vi "001_Faith FT6400 Series.vi"(11 "Queue Ref":T1={"UI"=refnum, "Message"=refnum, "Data"=refnum, "Caller"=refnum, "Name"="000 Common", "Data Path"=path "D:/NBT/01-Project/02-Processing/NBT-TestPlatform V2/NBT-TestPlatform V2.0.3/Config/NBT/NBT_V1.0.0/Project/0001_HZKD_ST01/00_DataSource/001_PLC/01_PLC", "Class Path"=path "", "SubPanel"=refnum, "Project Name"="", "MNT"="", "Title"="", "Data Source"=refnum, "Queue List"={}, "VI"=refnum, "UE"=refnum}) -> ()   [LabVIEW 2020]
doc: "000001"
uses:
  Alin/QMH/000 Module Data Type.ctl
  Alin/QMH/Queue Message.ctl
  0007 Controls/005 Data Source Type.ctl
  9999 SubVI/Global/Data Global/SDQ Data Type.ctl
  002 Driver/002 Electronic Load/Load Param.ctl
  c9d39cc7-6b3d-4d6b-ac97-2b41707d41b7.vi
panel:
  out "QN":i32
  in  "Panel Show":bool
  out "Data Type Out":T2
  in  "Panel Insert":bool
  out "Open":bool
  out "Model":string
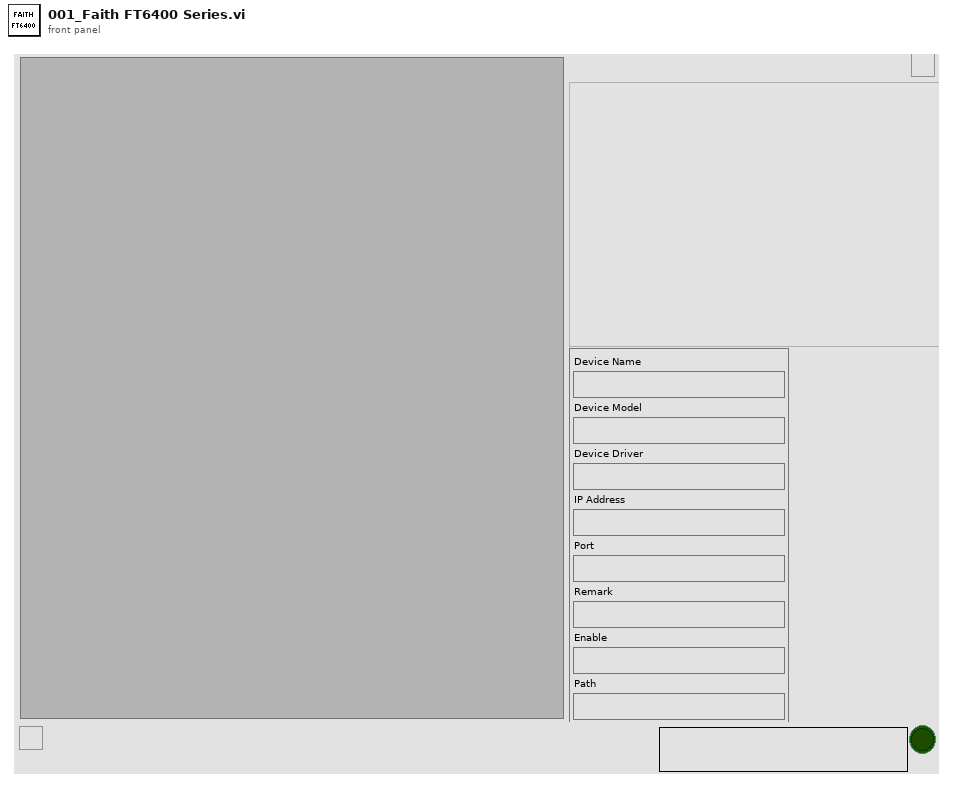
[diagram p1: front panel]
types:
  T1 = typedef "000 Module Data Type.ctl" = cluster{"UI":refnum<queue>, "Message":refnum<queue>, "Data":refnum<queue>, "Caller":refnum<queue>, "Name":string, "Data Path":path, "Class Path":path, "SubPanel":refnum<vi>, "Project Name":string, "MNT":string, "Title":string, "Data Source":refnum<queue>, "Queue List":map{string, refnum<queue>}, "VI":refnum<vi>, "UE":refnum<user-event>}
  T2 = typedef "005 Data Source Type.ctl" = cluster{"Device Name":string, "Device Model":string, "Device Driver":string, "IP Address":string, "Port":string, "Remark":string, "Enable":string, "Path":string}
  T3 = typedef "SDQ Data Type.ctl" = cluster{"CAN Length":string, "CAN Name":string, "CAN ID":string, "CAN Type":string, "Test Item":string, "Byte Order":string, "Instruction":string, "Control Type":string, "Group":string, "Offset":dbl, "Coefficient":dbl, "Write Enable":bool, "Lable Type":string, "Key?":string, "Set Value":string, "Upper":dbl, "Lower":dbl, "Unit":string, "Formula":string, "Test Item Type":string, "Length":i32, "Address":string, "Name":string, "Identifier":string, "Data Type":string, "Enumerate?":string, "Enumerate List":string, "Data":string, "Source":string}
  T4 = cluster{"Read":map{string, string}, "Open?":bool, "Start?":bool, "Queue Ref":T1, "Data":map{string, T3}, "Data List":T3[], "Data List02":cluster{"Identifier":string, "Name":string, "Data":string, "Unit":string}[], "Data Type Out":T2, "Visa":refnum<visa-resource-name>, "IDs":string, "Open?":bool}
  T5 = typedef "Load Param.ctl" = enum16{"Voltage", "Current", "Power", "Voltage_Set", "Current_Set", "Power_Set", "Mode", "Output", "Error"}
  T6 = cluster{"Name":string, "Read":map{string, string}}
  T7 = typedef "eventvkey.ctl" = enum16{"ASCII", "Enter", "Return", "Shift", "Ctrl", "Alt", "Cmd", "Opt", "Caps", "NumLock", "Clear", "Break", "Up", "Down", "Left", "Right", "Insert", "Delete", "Home", "End", "PageUp", "PageDown", "Escape", "Help", "Pause", "ScrollLock", "F1", "F2", "F3", "F4", "F5", "F6", "F7", "F8", "F9", "F10", "F11", "F12", "F13", "F14", "F15", "F16", "F17", "F18", "F19", "F20", "F21", "F22", "F23", "F24", "Play", "VolumeUp", "VolumeDown", "Mute", "Two Byte Char"}
  T8 = cluster{"Shift":bool, "Ctrl":bool, "Alt":bool, "Cmd":bool, "Opt":bool}
  T9 = cluster{"Queue List":map{string, refnum<queue>}, "Active Panel":string, "Queue Ref":T1, "SubPanel":refnum<vi>}
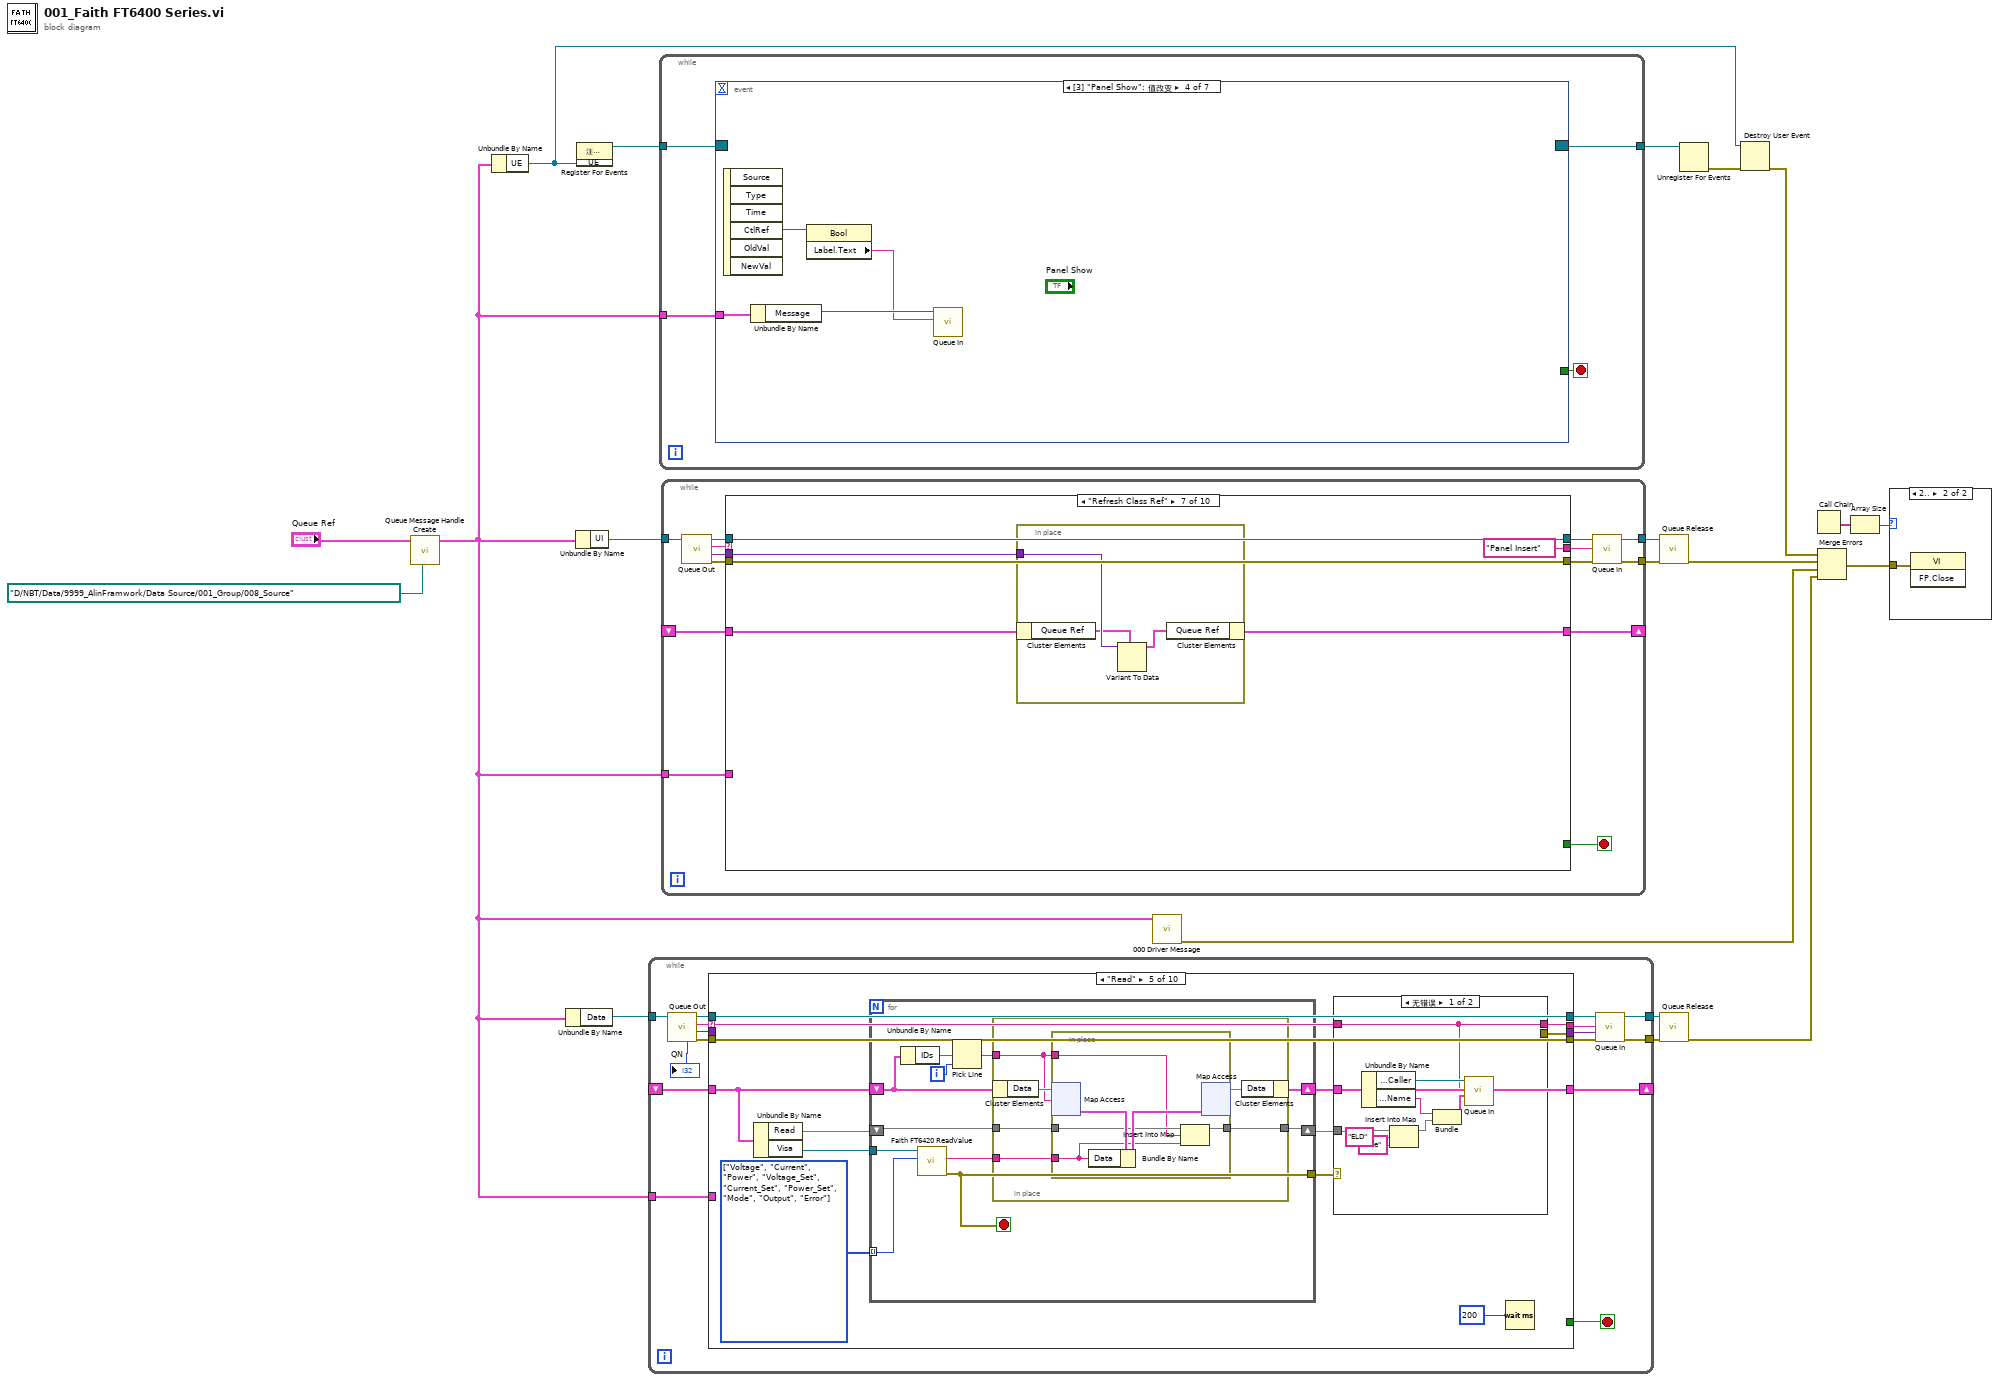
[diagram p0: block diagram]
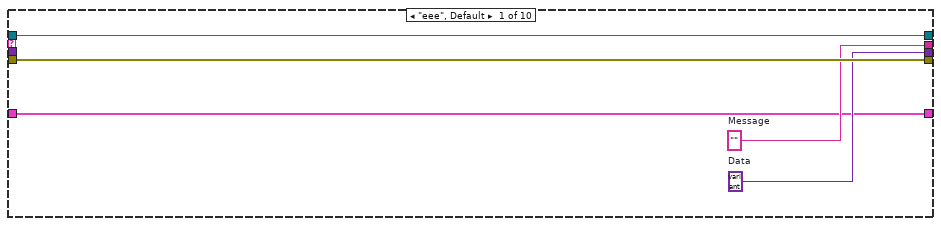
[diagram p2: hidden frame]
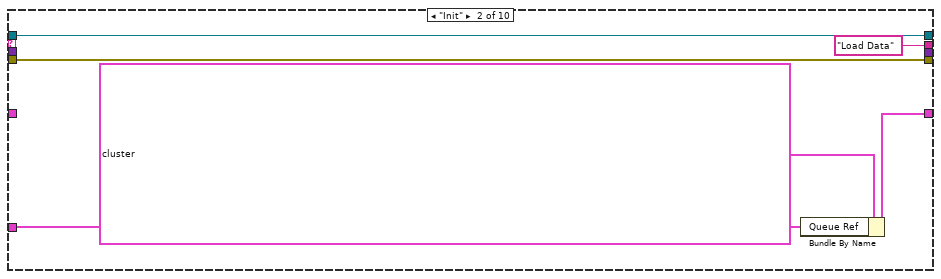
[diagram p3: hidden frame]
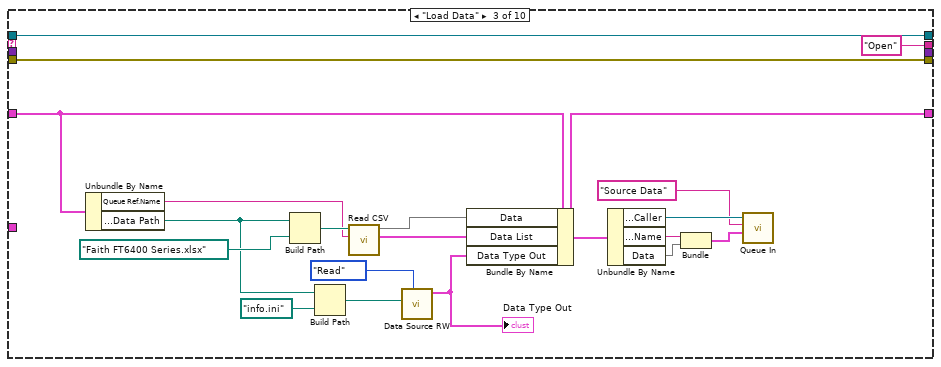
[diagram p4: hidden frame]
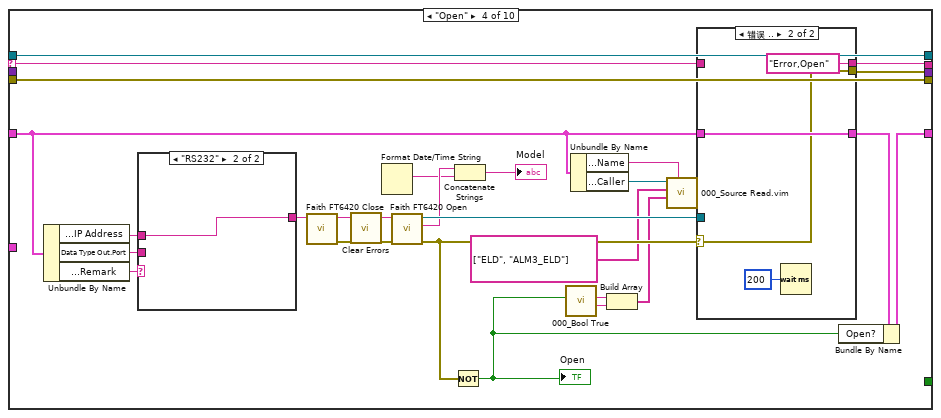
[diagram p5: hidden frame]
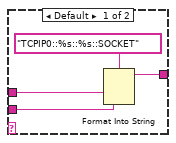
[diagram p6: hidden frame]
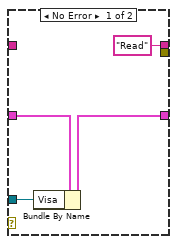
[diagram p7: hidden frame]
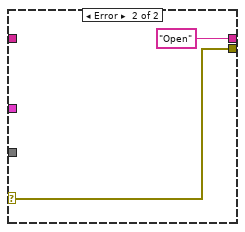
[diagram p8: hidden frame]
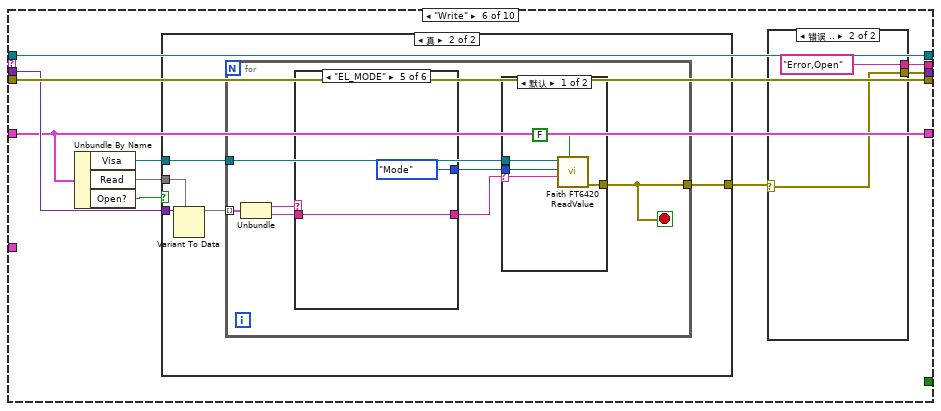
[diagram p9: hidden frame]
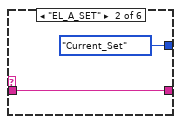
[diagram p13: hidden frame]
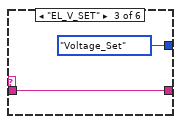
[diagram p14: hidden frame]
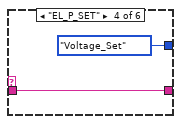
[diagram p15: hidden frame]
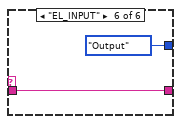
[diagram p16: hidden frame]
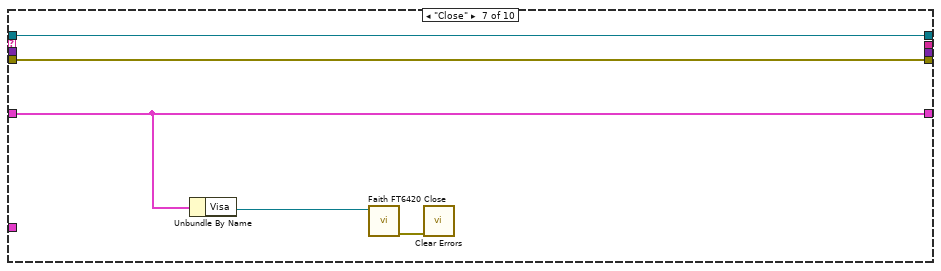
[diagram p18: hidden frame]
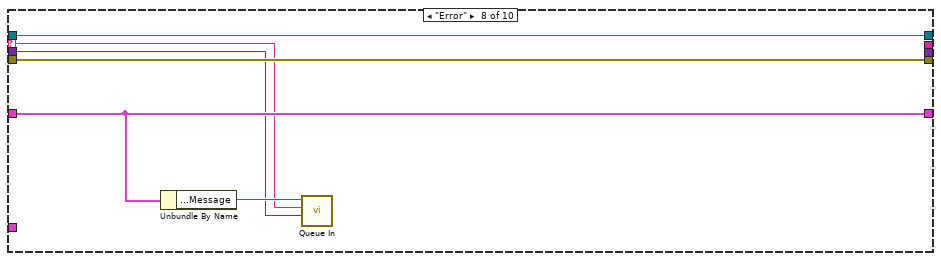
[diagram p19: hidden frame]
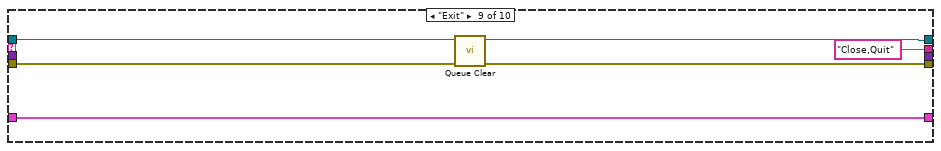
[diagram p20: hidden frame]
diagram:
  n1 = call "Queue Message Handle Create.vi"("Data Path"=path "D:/NBT/Data/9999_AlinFramwork/Data Source/001_Group/008_Source", "Queue Ref In"="Queue Ref") -> ("Queue Ref Out"=w3:T1)  [unwired: 8 in, 1 out]
  n2 = Unbundle By Name(w3) -> ("UE"=w2:refnum<user-event>)
  n3 = Unbundle By Name(w3) -> ("Data"=w18:refnum<queue>)
  n4 = Unbundle By Name(w3) -> ("UI"=w10:refnum<queue>)
  n5 = register-events(w2) -> (reference out=w5:refnum<event-registration>)  [unwired: 2 in, 1 out]
  n6 = while {
    tunnel: w18 -> [w32]
    tunnel: [w29] -> w16
    tunnel: [w28] -> w17
    shift-right: [w22] -> _
    shift-left: _ -> [w24]
    tunnel: w3 -> [w23]
    stop <- w36 stop-if-true
    n7 = call "Queue Out.vi"("Queue In"=w32) -> ("error out"=w35:errorcluster, "Data"=w33:variant, "Message"=w34:string, "Queue Out"=w31:refnum<queue>, "Queue NUmber"=→"QN":i32)  [unwired: 6 in]
    n8 = case shown="\"Read\"" w34 {
      selector: w34 -> [_ _ _ w82 w108 _ _ w199 _ _]
      tunnel: w31 -> [w41 w47 w67 w93 w119 w163 w197 w203 w208 w212]
      tunnel: w35 -> [w40 w46 w66 w92 w118 w162 w196 w202 w206 w213]
      tunnel: [w41 w47 w67 w93 w119 w163 w197 w203 w207 w212] -> w30
      tunnel: [w40 w46 w66 w92 w118 w162 w196 w202 w205 w213] -> w27
      tunnel: [w39 "Load Data" ("Message") "Open" ("Message") w81 w110 w155 _ _ "Close,Quit" _] -> w26
      tunnel: [_ _ _ _ _ _ _ _ _ TRUE] -> w36
      tunnel: [w38 _ _ w73 w107 w156 _ _ _ _] -> w25
      tunnel: w33 -> [_ _ _ _ _ w161 _ w198 _ _]
      tunnel: [w37 w44 w56 w69 w113 w159 w195 w200 w204 w210] -> w22
      tunnel: w24 -> [w37 _ w65 w80 w115 w159 w195 w200 w204 w210]
      tunnel: w23 -> [_ w43 _ _ _ _ _ _ _ _]
      frame "eee", Default {
        w38 = variant  # Data
        w39 = ""  # Message
      }
      frame "Init" {
        n9 = Bundle By Name(cluster=T4 {"Read"={}, "Open?"=FALSE, "Start?"=FALSE, "Queue Ref"={"UI"=refnum, "Message"=refnum, "Data"=refnum, "Caller"=refnum, "Name"="", "Data Path"=path "", "Class Path"=path "", "SubPanel"=refnum, "Project Name"="", "MNT"="", "Title"="", "Data Source"=refnum, "Queue List"={}, "VI"=refnum, "UE"=refnum}, "Data"={}, "Data List"=[], "Data List02"=[], "Data Type Out"={"Device Name"="费思负载", "Device Model"="Faith Load", "Device Driver"="Faith Load", "IP Address"="192.168.0.178", "Port"="7001", "Remark"="TCP", "Enable"="True", "Path"="004_Source"}, "Visa"="", "IDs"="EL_V\nEL_A\nEL_P\nEL_V_SET\nEL_A_SET\nEL_P_SET\nEL_MODE\nEL_INPUT\nEL_ERROR", "Open?"=FALSE}, "Queue Ref"=w43) -> (w44:T4)
      }
      frame "Load Data" {
        n10 = Unbundle By Name(w65) -> ("Queue Ref.Name"=w54:string, "Queue Ref.Data Path"=w52:path)
        n11 = Build Path(base path=w52, name or relative path=path "Faith FT6400 Series.xlsx" ("名称或相对路径")) -> (appended path=w64:path)
        n12 = Build Path(base path=w52, name or relative path=path "info.ini" ("名称或相对路径")) -> (appended path=w50:path)
        n13 = call "Read CSV.vi"("Source"=w54, "Data Path"=w64) -> ("Identifier List"=w62:T3[], "Identifiers Out"=w61:map{string, T3})  [unwired: 2 in, 6 out]
        n14 = call "Data Source RW.vi"("Operate"=enum16{"Read", "Write"}."Read", "Source Path"=w50) -> ("Data Type Out"=w48:T2)  [unwired: 6 in, 3 out]
        "Data Type Out" <- w48
        n15 = Bundle By Name(cluster=w65, "Data"=w61, "Data List"=w62, "Data Type Out"=w48) -> (w56:T4)
        n16 = Unbundle By Name(w56) -> ("Queue Ref.Caller"=w57:refnum<queue>, "Queue Ref.Name"=w60:string, "Data"=w58:map{string, T3})
        n17 = Bundle("Name"=w60, "Data"=w58) -> (w59:cluster{"Name":string, "Data":map{string, T3}})  [unwired: 1 in]
        n18 = call "Queue In.vi"("Data"=w59, "Message"="Source Data", "Queue In"=w57) -> ()  [unwired: 7 in, 2 out]
      }
      frame "Open" {
        n19 = Unbundle By Name(w80) -> ("Data Type Out.IP Address"=w91:string, "Data Type Out.Port"=w90:string, "Data Type Out.Remark"=w70:string)
        n20 = case shown="\"RS232\"" w70 {
          tunnel: w91 -> [w96 w98]
          tunnel: w90 -> [w95 _]
          tunnel: [w94 w98] -> w72
          frame Default {
            n21 = Format Into String(format string="TCPIP0::%s::%s::SOCKET" ("格式字符串"), w96, w95) -> (resulting string=w94:string)  [unwired: 2 in, 1 out]
          }
          frame "RS232" {
          }
        }
        n22 = call "Faith FT6420 Close.vi"("visa in"=w72) -> ("error out"=w71:errorcluster)  [unwired: 10 in]
        n23 = call <vilib>:"Clear Errors.vi"("error in (no error)"=w71) -> ("error out"=w83:errorcluster)  [unwired: 5 in, 1 out]
        n24 = Format Date/Time String() -> (date/time string=w85:string)  [unwired: 3 in]
        n25 = call "Faith FT6420 Open.vi"("error in (no error)"=w83, "visa in"=w72) -> ("error out"=w87:errorcluster, "Modle"=w86:string, "visa out"=w88:refnum<visa-resource-name>)  [unwired: 7 in]
        n26 = Not(x=w87) -> (.not. x?=w68:bool)
        "Open" <- w68
        n27 = Concatenate Strings(w86, w85) -> (→"Model":string)
        n28 = call "000_Bool True.vi"("Value"=w68) -> ("Anti"=w75:string, "String Out"=w76:string)  [unwired: 8 in, 1 out]
        n29 = Unbundle By Name(w80) -> ("Queue Ref.Name"=w78:string, "Queue Ref.Caller"=w79:refnum<queue>)
        n30 = Build Array(w76, w75) -> (w74:string[])
        n31 = call "000_Source Read.vim"("Surce"=w78, "Data"=w74, "Name"=string[] ["ELD", "ALM3_ELD"], "Queue In"=w79) -> ()  [unwired: 5 in, 3 out]
        n32 = case shown="错误 .." w87 {
          selector: w87 -> [_ w103]
          tunnel: w80 -> [w102 w106]
          tunnel: [w101 w106] -> w89
          tunnel: w88 -> [w100 _]
          tunnel: w82 -> [_ _]
          tunnel: ["Read" "Error,Open"] -> w81
          tunnel: [_ w103] -> w73
          frame No Error {
            n33 = Bundle By Name(cluster=w102, "Visa"=w100) -> (w101:T4)
          }
          frame Error {
            n34 = Wait (ms)(milliseconds to wait=u32 200 ("等待时间（毫秒）")) -> ()  [unwired: 1 out]
          }
        }
        n35 = Bundle By Name(cluster=w89, "Open?"=w68) -> (w69:T4)
      }
      frame "Read" {
        w116 = T5[] [enum."Voltage", enum."Current", enum."Power", enum."Voltage_Set", enum."Current_Set", enum."Power_Set", enum."Mode", enum."Output", enum."Error"] items=["Voltage", "Current", "Power", "Voltage_Set", "Current_Set", "Power_Set", "Mode", "Output", "Error"] ("数组")
        n36 = Unbundle By Name(w115) -> ("Read"=w114:map{string, string}, "Visa"=w117:refnum<visa-resource-name>)
        n37 = for {
          tunnel: w117 -> [w141]
          tunnel: w116 -> [w140] mode=indexing
          shift-right: [w139] -> w113
          shift-left: w115 -> [w138]
          shift-right: [w132] -> w112
          shift-left: w114 -> [w133]
          tunnel: [w131] -> w111
          i -> [w136]
          stop <- w131 stop-if-true
          n38 = Unbundle By Name(w138) -> ("IDs"=w137:string)
          n39 = call "Faith FT6420 ReadValue.vi"("Mode"=w140, "visa in"=w141) -> ("error out"=w131:errorcluster, "Value Out"=w134:string)  [unwired: 6 in, 2 out]
          n40 = Pick Line(multi-line string=w137, line index=w136) -> (output string=w135:string)  [unwired: 1 in]
          n41 = in-place {
            in-place-border: w135 -> [w143]
            in-place-border: w134 -> [w145]
            in-place-border: w133 -> [w144]
            in-place-border: [w142] -> w132
            n42 = in-place-cluster #1(w138) -> ("Data"=w147:map{string, T3})
            n43 = in-place {
              in-place-border: w145 -> [w149]
              in-place-border: w144 -> [w151]
              in-place-border: w143 -> [w150]
              in-place-border: [w148] -> w142
              n44 = in-place-map #2(w147, w143) -> (w153:T3)  [unwired: 1 in, 1 out]
              n45 = Bundle By Name(cluster=w153, "Data"=w149) -> (w152:T3)
              n46 = Insert Into Map(map in=w151, key=w150, value=w149) -> (map out=w148:map{string, string})  [unwired: 2 out]
              n47 = in-place-map #2(w152) -> (w146:map{string, T3})  [unwired: 1 in, 2 out]
            }
            n48 = in-place-cluster #1("Data"=w146) -> (w139:T4)
          }
        }
        n49 = case shown="无错误" w111 {
          selector: w111 -> [_ w129]
          tunnel: w113 -> [w127 _]
          tunnel: w112 -> [w123 _]
          tunnel: [w124 "Open"] -> w110
          tunnel: w108 -> [w124 _]
          tunnel: [_ w129] -> w107
          frame No Error {
            n50 = Unbundle By Name(w127) -> ("Queue Ref.Caller"=w126:refnum<queue>, "Queue Ref.Name"=w125:string)
            n51 = Insert Into Map(map in=w123, key="ELD" ("键"), value="true" ("值")) -> (map out=w122:map{string, string})  [unwired: 2 out]
            n52 = Bundle("Name"=w125, "Read"=w122) -> (w128:T6)  [unwired: 1 in]
            n53 = call "Queue In.vi"("Data"=w128, "Message"=w124, "Queue In"=w126) -> ()  [unwired: 7 in, 2 out]
          }
          frame Error {
          }
        }
        n54 = Wait (ms)(milliseconds to wait=u32 200 ("等待时间（毫秒）")) -> ()  [unwired: 1 out]
      }
      frame "Write" {
        n55 = Unbundle By Name(w159) -> ("Visa"=w158:refnum<visa-resource-name>, "Read"=w160:map{string, string}, "Open?"=w154:bool)
        n56 = case shown="真" w154 {
          tunnel: w161 -> [_ w168]
          tunnel: w160 -> [_ w167]
          tunnel: w158 -> [_ w165]
          tunnel: [_ w164] -> w157
          frame False {
          }
          frame True {
            n57 = Variant To Data(type=w167, Variant=w168) -> (data=w166:map{string, string})  [unwired: 1 in, 1 out]
            n58 = for {
              tunnel: w166 -> [w175] mode=indexing
              tunnel: w165 -> [w173]
              tunnel: [w171] -> w164
              stop <- w171 stop-if-true
              n59 = Unbundle(w175) -> ("Identifier"=w174:string, "Data"=w172:string)
              n60 = case shown="\"EL_MODE\"" w174 {
                tunnel: w172 -> [_ w181 w183 w185 w187 w189]
                tunnel: [_ Load_Param."Current_Set" ("Mode") Load_Param."Voltage_Set" ("Mode") Load_Param."Voltage_Set" ("Mode") Load_Param."Mode" ("Mode") Load_Param."Output" ("Mode")] -> w170
                tunnel: [_ w181 w183 w185 w187 w189] -> w169
                frame Default {
                }
                frame "EL_A_SET" {
                }
                frame "EL_V_SET" {
                }
                frame "EL_P_SET" {
                }
                frame "EL_MODE" {
                }
                frame "EL_INPUT" {
                }
              }
              n61 = case shown="默认" w169 {
                selector: w169 -> [w176 _]
                tunnel: w173 -> [w179 _]
                tunnel: [w178 _] -> w171
                tunnel: w170 -> [w177 _]
                frame Default {
                  n62 = call "Faith FT6420 ReadValue.vi"("Query?"=FALSE, "Value In"=w176, "Mode"=w177, "visa in"=w179) -> ("error out"=w178:errorcluster)  [unwired: 4 in, 3 out]
                }
                frame "" {
                }
              }
            }
          }
        }
        n63 = case shown="错误 .." w157 {
          selector: w157 -> [_ w192]
          tunnel: [_ w192] -> w156
          tunnel: [_ "Error,Open"] -> w155
          frame No Error {
          }
          frame Error {
          }
        }
      }
      frame "Close" {
        n64 = Unbundle By Name(w195) -> ("Visa"=w194:refnum<visa-resource-name>)
        n65 = call "Faith FT6420 Close.vi"("visa in"=w194) -> ("error out"=w193:errorcluster)  [unwired: 10 in]
        n66 = call <vilib>:"Clear Errors.vi"("error in (no error)"=w193) -> ()  [unwired: 5 in, 2 out]
      }
      frame "Error" {
        n67 = Unbundle By Name(w200) -> ("Queue Ref.Message"=w201:refnum<queue>)
        n68 = call "Queue In.vi"("Data"=w198, "Message"=w199, "Queue In"=w201) -> ()  [unwired: 7 in, 2 out]
      }
      frame "Exit" {
        n69 = call "Queue Clear.vi"("error in (no error)"=w206, "Queue In"=w208) -> ("error out"=w205:errorcluster, "Queue Out"=w207:refnum<queue>)  [unwired: 8 in]
      }
      frame "Quit" {
      }
    }
    n70 = call "Queue In.vi"("error in (no error)"=w27, "Data"=w25, "Message"=w26, "Queue In"=w30) -> ("error out"=w28:errorcluster, "Queue Out"=w29:refnum<queue>)  [unwired: 6 in]
  }
  n71 = while {
    tunnel: w5 -> [w217]
    tunnel: [w215] -> w6
    tunnel: w3 -> [w214]
    stop <- w216 stop-if-true
    n72 = event shown="[3] \"Panel Show\": 值改变" {
      selector: w217 -> [_ _ _ _ _ _ _]
      dyn-events: [_ _ _ _ _ _ _] -> w215
      timeout: _ -> [_ _ _ _ _ _ _]
      tunnel: [_ _ _ _ _ w234 _] -> w216
      tunnel: w214 -> [_ w222 w226 w230 w233 _ w238]
      event Timeout {
        n73 = event-data() -> ()  [unwired: 1 in, 1 out]
      }
      event Key Down {
        n74 = event-data() -> ("Char"=w221:i16, "VKey"=w220:T7, "Mods"=w219:cluster{"Num Pad":bool, "Menu Key":bool}, "PlatMods"=w218:T8)  [unwired: 1 in]
        n75 = call "Queue Key Down.vi"("Queue Ref Out"=w222, "C"=w221, "Platform Key"=w218, "Group Key"=w219, "V Key"=w220) -> ()  [unwired: 6 in, 1 out]
      }
      event "Panel Insert": Value Change {
        n76 = event-data() -> ("CtlRef"=w224:refnum<vi>)  [unwired: 1 in, 5 out]
        n77 = Unbundle By Name(w226) -> ("UI"=w225:refnum<queue>)
        n78 = property class="Bool"(reference=w224) -> ("Label.Text"=w223:string)  [unwired: 1 in, 2 out]
        n79 = call "Queue In.vi"("Message"=w223, "Queue In"=w225) -> ()  [unwired: 8 in, 2 out]
      }
      event "Panel Show": Value Change {
        n80 = event-data() -> ("CtlRef"=w228:refnum<vi>)  [unwired: 1 in, 5 out]
        n81 = Unbundle By Name(w230) -> ("Message"=w229:refnum<queue>)
        n82 = property class="Bool"(reference=w228) -> ("Label.Text"=w227:string)  [unwired: 1 in, 2 out]
        n83 = call "Queue In.vi"("Message"=w227, "Queue In"=w229) -> ()  [unwired: 8 in, 2 out]
      }
      event Panel Resize {
        n84 = event-data() -> ()  [unwired: 1 in, 1 out]
        n85 = Unbundle By Name(w233) -> ("Message"=w232:refnum<queue>)
        n86 = call "Queue In.vi"("Message"="Panel Change", "Queue In"=w232) -> ()  [unwired: 8 in, 2 out]
      }
      event User Event {
        n87 = event-data() -> ("Message"=w236:string)  [unwired: 1 in]
        n88 = Equal?(x=w236, y="Exit") -> (x = y?=w234:bool)
      }
      event Panel Close? {
        n89 = event-data() -> ()  [unwired: 1 in, 1 out]
        n90 = Unbundle By Name(w238) -> ("Message"=w237:refnum<queue>)
        n91 = Call Chain() -> (call chain=w241:string[])
        n92 = Array Size(array=w241) -> (size(s)=w240:i32)
        n93 = case shown="0, 默认" w240 {
          tunnel: ["Exit Prepare" ("Message") "Panel Hidden" ("Message")] -> w239
          frame 0, Default {
          }
          frame 2.. {
          }
        }
        n94 = call "Queue In.vi"("Message"=w239, "Queue In"=w237) -> ()  [unwired: 8 in, 2 out]
        n95 = event-data("Discard?"=TRUE ("放弃？")) -> ()  [unwired: 1 in, 1 out]
      }
    }
  }
  n96 = while {
    tunnel: w10 -> [w254]
    tunnel: [w251] -> w8
    tunnel: [w250] -> w9
    tunnel: w3 -> [w247]
    shift-right: [w246] -> _
    shift-left: _ -> [w245]
    stop <- w258 stop-if-true
    n97 = call "Queue Out.vi"("Queue In"=w254) -> ("error out"=w257:errorcluster, "Data"=w255:variant, "Message"=w256:string, "Queue Out"=w253:refnum<queue>)  [unwired: 6 in, 1 out]
    n98 = case shown="\"Refresh Class Ref\"" w256 {
      selector: w256 -> [_ _ _ w291 _ w304 _ _ w323 _]
      tunnel: w253 -> [w261 w268 w286 w295 w301 w308 w314 w320 w330 w337]
      tunnel: w257 -> [w260 w267 w285 w294 w300 w307 w313 w319 w328 w338]
      tunnel: [w261 w268 w286 w295 w301 w308 w314 w320 w329 w337] -> w252
      tunnel: [w260 w267 w285 w294 w300 w307 w313 w319 w327 w338] -> w249
      tunnel: [_ "Launch DataMinitor" _ _ _ _ "Panel Insert" _ "Quit" _] -> w248
      tunnel: [_ _ _ _ _ _ _ _ _ TRUE] -> w258
      tunnel: w255 -> [_ _ _ _ _ _ w310 _ _ _]
      tunnel: w247 -> [_ w264 _ _ _ w306 _ _ _ _]
      tunnel: [w259 w265 w284 w293 w299 w303 w311 w318 w322 w335] -> w246
      tunnel: w245 -> [w259 _ w284 w293 w299 w303 w312 w318 w322 w335]
      frame "eee", Default {
      }
      frame "Init" {
        n99 = control-ref of="SubPanel"() -> (w263:refnum<vi>)
        n100 = Bundle By Name(cluster=T9 {"Queue List"={}, "Active Panel"="", "Queue Ref"={"UI"=refnum, "Message"=refnum, "Data"=refnum, "Caller"=refnum, "Name"="", "Data Path"=path "", "Class Path"=path "", "SubPanel"=refnum, "Project Name"="", "MNT"="", "Title"="", "Data Source"=refnum, "Queue List"={}, "VI"=refnum, "UE"=refnum}, "SubPanel"=refnum}, "Queue Ref"=w264, "SubPanel"=w263) -> (w265:T9)
      }
      frame "Launch DataMinitor" {
        w269 = "DataMonitor" ("格式字符串")
        n101 = vi-ref "002_DataMonitor.vi"() -> (w281:refnum<vi>)
        n102 = property class="VI"(reference=w281) -> ("Path"=w280:path)  [unwired: 1 in, 2 out]
        n103 = Unbundle By Name(w284) -> ("Queue Ref"=w283:T1, "SubPanel"=w282:refnum<vi>, "Queue Ref.Data Path"=w279:path, "Queue Ref.Name"=w270:string)
        n104 = Build Path(base path=w279, name or relative path=w269) -> (appended path=w278:path)
        n105 = call <vilib>:"Check if File or Folder Exists.vi"("path"=w278) -> ("error out"=w276:errorcluster, "file or folder exists?"=w277:bool, "dup path"=w275:path)  [unwired: 8 in]
        n106 = case shown="真" w277 {
          tunnel: w276 -> [w289 _]
          tunnel: w275 -> [w288 w290]
          tunnel: [w287 w290] -> w274
          frame False {
            n107 = Create Folder(path (use dialog)=w288, error in=w289) -> (created path=w287:path)  [unwired: 1 in, 2 out]
          }
          frame True {
          }
        }
        n108 = Format Into String(format string="%s_%s" ("格式字符串"), w270, w269) -> (resulting string=w271:string)  [unwired: 2 in, 1 out]
        n109 = Bundle By Name(cluster=w283, "SubPanel"=w282, "Class Path"=w280, "Data Path"=w274, "Name"=w271) -> (w273:T1)
        n110 = call "000 Client Launch.vi"("Queue Ref"=w273) -> ()  [unwired: 10 in, 1 out]
      }
      frame "Panel Insert" {
        n111 = Unbundle By Name(w293) -> ("Queue Ref.Queue List"=w292:map{string, refnum<queue>})
        n112 = for {
          tunnel: w292 -> [w298] mode=indexing
          tunnel: w291 -> [w296]
          n113 = Unbundle(w298) -> ("Client Refer"=w297:refnum<queue>)  [unwired: 1 out]
          n114 = call "Queue In.vi"("Message"=w296, "Queue In"=w297) -> ()  [unwired: 8 in, 2 out]
        }
      }
      frame "====System====" {
      }
      frame "Client Delete", "Client Launch" {
        n115 = Unbundle By Name(w306) -> ("Message"=w305:refnum<queue>)
        n116 = Unbundle By Name(w303) -> ("Active Panel"=w302:string)
        n117 = call "Queue In.vi"("Data"=w302, "Message"=w304, "Queue In"=w305) -> ()  [unwired: 7 in, 2 out]
      }
      frame "Refresh Class Ref" {
        n118 = in-place {
          in-place-border: w310 -> [w317]
          n119 = in-place-cluster #3(w312) -> ("Queue Ref"=w316:T1)
          n120 = Variant To Data(type=w316, Variant=w317) -> (data=w315:T1)  [unwired: 1 in, 1 out]
          n121 = in-place-cluster #3("Queue Ref"=w315) -> (w311:T9)
        }
      }
      frame "====User====" {
      }
      frame "Exit" {
        n122 = Unbundle By Name(w322) -> ("Queue Ref.UE"=w321:refnum<user-event>, "Queue Ref.Message"=w326:refnum<queue>, "Queue Ref.Data"=w325:refnum<queue>)
        n123 = Build Array(w326, w325) -> (w324:refnum<queue>[])
        n124 = Generate User Event(user event=w321, event data cluster=w323) -> ()  [unwired: 2 in, 2 out]
        n125 = for {
          tunnel: w324 -> [w334] mode=indexing
          tunnel: w323 -> [w333]
          n126 = call "Queue In.vi"("First"=TRUE, "Message"=w333, "Queue In"=w334) -> ()  [unwired: 7 in, 2 out]
        }
        n127 = call "Queue Clear.vi"("error in (no error)"=w328, "Queue In"=w330) -> ("error out"=w327:errorcluster, "Queue Out"=w329:refnum<queue>)  [unwired: 8 in]
      }
      frame "Quit" {
      }
    }
    n128 = call "Queue In.vi"("error in (no error)"=w249, "Message"=w248, "Queue In"=w252) -> ("error out"=w250:errorcluster, "Queue Out"=w251:refnum<queue>)  [unwired: 7 in]
  }
  n129 = call "000 Driver Message.vi"("Queue In"=w3) -> ("error out"=w19:errorcluster)  [unwired: 8 in, 2 out]
  n130 = call "Queue Release.vi"("error in (no error)"=w9, "Queue In"=w8) -> ("error out"=w12:errorcluster)  [unwired: 9 in]
  n131 = call "Queue Release.vi"("error in (no error)"=w17, "Queue In"=w16) -> ("error out"=w20:errorcluster)  [unwired: 9 in]
  n132 = Unregister For Events(event registration refnum=w6) -> (error out=w7:errorcluster)  [unwired: 1 in]
  n133 = Destroy User Event(user event=w2, error in=w7) -> (error out=w11:errorcluster)
  n134 = Call Chain() -> (call chain=w14:string[])
  n135 = Merge Errors(w11, w12, w19, w20) -> (w13:errorcluster)
  n136 = Array Size(array=w14) -> (size(s)=w15:i32)
  n137 = case shown="2.." w15 {
    tunnel: w13 -> [_ w339]
    frame 0, Default {
    }
    frame 2.. {
      n138 = invoke class="VI" method="FP.Close"(error in=w339) -> ()  [unwired: 2 in, 3 out]
    }
  }
